vi "Gpad Drive 2898.vi"(7 "Right Side?":bool, 8 "Fire?":bool, 9 "Turn?":bool) -> (0 "Viewer Select":T1(ring)=enum."Ball Camera", 1 "Bridge Mode?":bool, 2 "Tank?":bool, 3 "Aligned?":bool, 5 "Shooter Is Front":bool)   [LabVIEW 2011]
uses:
  Team Code/Robot Global Data.vi
panel:
  in  "Bridge Mode Speed Reduction":dbl=2.0
  in  "Power Factor":dbl=3.0
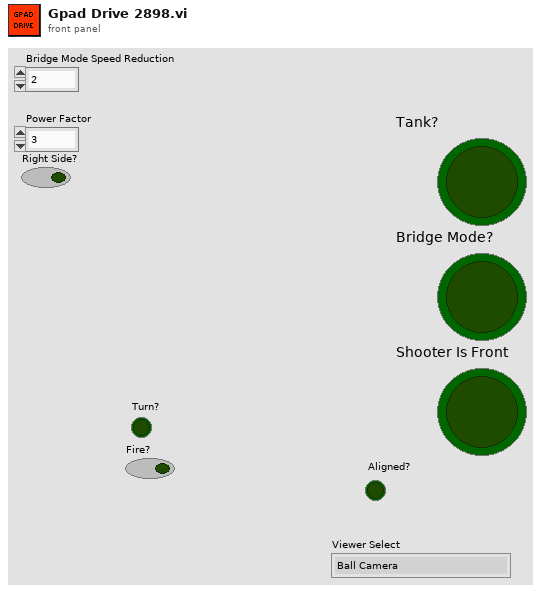
[diagram p1: front panel]
types:
  T1 = enum32{"Target Camera", "Target Camera Mask", "Ball Camera", "Kinect Skeleton"}
  T2 = typedef "WPI_JoystickButtonState.ctl" = cluster{"Button 1":bool, "Button 2":bool, "Button 3":bool, "Button 4":bool, "Button 5":bool, "Button 6":bool, "Button 7":bool, "Button 8":bool, "Button 9":bool, "Button 10":bool, "Button 11":bool, "Button 12":bool}
  T3 = cluster{"Buttons":T2, "Axes":cluster{"axis 1 (x)":dbl, "axis 2 (y)":dbl, "axis 3 (throttle)":dbl, "axis 4":dbl, "axis 5":dbl, "axis 6":dbl}}
  T4 = cluster{"Position":cluster{"X Angle":dbl, "Raw Y":dbl, "Raw X":dbl}, "Distance (ft)":dbl, "BB Angle":dbl}
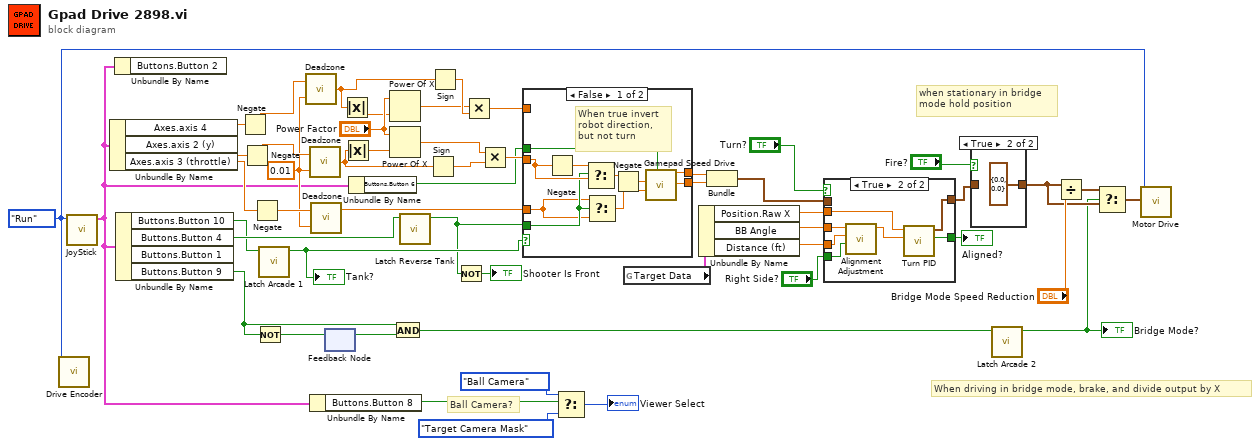
[diagram p0: block diagram]
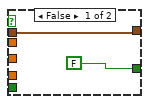
[diagram p3: hidden frame]
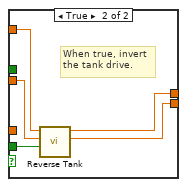
[diagram p4: hidden frame]
diagram:
  w13 = enum16{"Init", "Run", "End"}."Run" ("Enum")
  w46 = 0.01 ("Deadzone")
  # "Ball Camera?"
  # "when stationary in bridge \nmode hold position"
  # "When driving in bridge mode, brake, and divide output by X"
  n1 = call "Drive Encoder.vi"("Enum"=w13) -> ()  [unwired: 10 in, 1 out]
  n2 = call "JoyStick.vi"("Enum"=w13) -> ("JoyStick 1"=w22:T3)  [unwired: 7 in, 3 out]
  n3 = Unbundle By Name(w22) -> ("Axes.axis 4"=w48:dbl, "Axes.axis 2 (y)"=w50:dbl, "Axes.axis 3 (throttle)"=w51:dbl)
  n4 = Unbundle By Name(w22) -> ()  [unwired: 1 out]
  n5 = Unbundle By Name(w22) -> ("Buttons.Button 10"=w1:bool, "Buttons.Button 4"=w2:bool, "Buttons.Button 9"=w23:bool)  [unwired: 1 out]
  n6 = Negate(x=w48) -> (-x=w47:dbl)
  n7 = Negate(x=w50) -> (-x=w52:dbl)
  n8 = Negate(x=w51) -> (-x=w49:dbl)
  n9 = Not(x=w23) -> (.not. x?=w45:bool)
  n10 = call "Latch Arcade 1.vi"("Input"=w1) -> ("Latched"=w20:bool)  [unwired: 10 in]
  "Tank?" <- w20
  n11 = call "Deadzone.vi"("Deadzone"=w46, "Input"=w47) -> ("Output"=w11:dbl)
  n12 = call "Deadzone.vi"("Deadzone"=w46, "Input"=w52) -> ("Output"=w37:dbl)
  n13 = Unbundle By Name(w22) -> ("Buttons.Button 8"=w25:bool)
  n14 = call "Deadzone.vi"("Deadzone"=w46, "Input"=w49) -> ("Output"=w35:dbl)
  n15 = feedback-in #1(w45) -> ()
  n16 = feedback #1() -> (w44:bool)  [unwired: 1 in]
  n17 = Absolute Value(x=w11) -> (abs(x)=w10:dbl)
  n18 = Absolute Value(x=w37) -> (abs(x)=w9:dbl)
  n19 = Unbundle By Name(w22) -> ("Buttons.Button 6"=w36:bool)
  n20 = Power Of X(1:w10, 2:"Power Factor") -> (0:w8:dbl)
  n21 = Power Of X(1:w9, 2:"Power Factor") -> (0:w7:dbl)
  n22 = And(x=w23, y=w44) -> (x .and. y?=w21:bool)
  n23 = call "Latch Reverse Tank.vi"("Input"=w2) -> ("Latched"=w19:bool)  [unwired: 10 in]
  n24 = Sign(1:w37) -> (0:w38:dbl)
  n25 = Sign(1:w11) -> (0:w39:dbl)
  n26 = Not(x=w19) -> (.not. x?=→"Shooter Is Front":bool)
  n27 = Multiply(x=w8, y=w39) -> (x*y=w41:dbl)
  n28 = Multiply(x=w7, y=w38) -> (x*y=w40:dbl)
  n29 = case shown="False" w20 {
    tunnel: w36 -> [w59 _]
    tunnel: w40 -> [w57 w67]
    tunnel: w35 -> [w55 _]
    tunnel: [w62 w66] -> w34
    tunnel: [w61 w63] -> w33
    tunnel: w19 -> [w56 w65]
    tunnel: w41 -> [_ w64]
    frame False {
      # "When true invert robot direction, but not turn"
      n30 = Negate(x=w57) -> (-x=w58:dbl)
      n31 = Select(t=w58, s=w56, f=w57) -> (s? t:f=w54:dbl)
      n32 = Select(t=w55, s=w56, f=w55) -> (s? t:f=w60:dbl)
      n33 = Negate(x=w54) -> (-x=w53:dbl)
      n34 = call "Gamepad Speed Drive.vi"("Quick Turn"=w59, "Turn"=w60, "Speed"=w53) -> ("Right Output"=w61:dbl, "Left Output"=w62:dbl)  [unwired: 7 out]
    }
    frame True {
      # "When true, invert\nthe tank drive."
      n35 = call "Reverse Tank.vi"("Toggle Button"=w65, "Right Motor"=w67, "Left Motor"=w64) -> ("Right Motor"=w63:dbl, "Left Motor"=w66:dbl)  [unwired: 7 in]
    }
  }
  n36 = Select(t=T1."Ball Camera" ("Viewer Select"), s=w25, f=T1."Target Camera Mask" ("Viewer Select")) -> (s? t:f=→"Viewer Select":T1)
  n37 = global read "Robot Global Data.vi" "Target Data"() -> (w17:T4)
  n38 = Unbundle By Name(w17) -> ("Position.Raw X"=w31:dbl, "BB Angle"=w30:dbl, "Distance (ft)"=w29:dbl)
  n39 = Bundle("Left Motor"=w34, "Right Motor"=w33) -> (w15:cluster{"Left Motor":dbl, "Right Motor":dbl})  [unwired: 1 out]
  n40 = case shown="True" "Turn?" {
    tunnel: [w69 w73] -> w18
    tunnel: w15 -> [w69 _]
    tunnel: w31 -> [_ w70]
    tunnel: [FALSE w72] -> w32
    tunnel: "Right Side?" -> [_ w76]
    tunnel: w29 -> [_ w75]
    tunnel: w30 -> [_ w74]
    frame False {
    }
    frame True {
      n41 = call "Alignment Adjustment.vi"("Right Side of Field?"=w76, "Distance"=w75, "BB Angle"=w74) -> ("X Setpoint"=w71:dbl)  [unwired: 8 in]
      n42 = call "Turn PID.vi"("Setpoint X"=w71, "Current X"=w70) -> ("Aligned?"=w72:bool, "Motor Out"=w73:cluster{"output":dbl, dbl})  [unwired: 8 in]
    }
  }
  "Aligned?" <- w32
  n43 = case shown="True" "Fire?" {
    tunnel: w18 -> [w77 _]
    tunnel: [w77 cluster{"output":dbl, dbl} {"output"=0.0, 0.0} ("Motor Out")] -> w5
    frame False {
    }
    frame True {
    }
  }
  n44 = call "Latch Arcade 2.vi"("Input"=w21) -> ("Latched"=w4:bool)  [unwired: 10 in]
  "Bridge Mode?" <- w4
  n45 = Divide(x=w5, y="Bridge Mode Speed Reduction") -> (x/y=w6:cluster{"output":dbl, "Right Motor":dbl})
  n46 = Select(t=w6, s=w4, f=w5) -> (s? t:f=w3:cluster{"output":dbl, "Right Motor":dbl})
  n47 = call "Motor Drive.vi"("Motor Input"=w3, "Enum"=w13) -> ()  [unwired: 10 in]
